vi "Iso Measurement Write.vi"(8 "error in":errorcluster, 10 "Iso Measurement STS":i32, 11 "Iso Measurement in":refnum<class "Iso Measurement.lvclass">) -> (0 "error out":errorcluster, 3 "Iso Measurement out":refnum<class "Iso Measurement.lvclass">)   [LabVIEW 2023, in "Iso Measurement.lvclass"]
uses:
  Iso Measurement.lvclass
  <vilib>/ADAS Replay HIL/Channels/Tag Wrapper/Tag Wrapper.lvlib
  <vilib>/ADAS Replay HIL/Channels/Tag Wrapper/Polymorphic/Write Channel (I32).vi
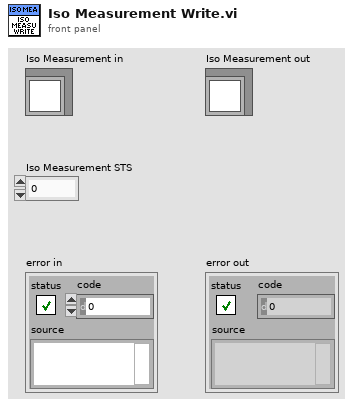
[diagram p1: front panel]
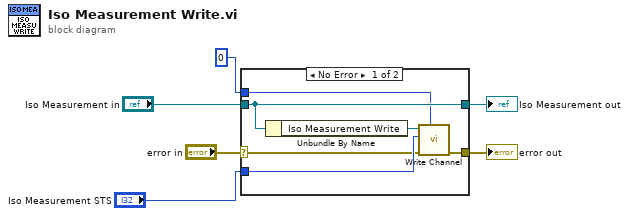
[diagram p0: block diagram]
diagram:
  n1 = case shown="No Error" "error in" {
    selector: "error in" -> [w9 w14]
    tunnel: [w8 w14] -> w5
    tunnel: [w12 w13] -> w3
    tunnel: "Iso Measurement in" -> [w12 w13]
    tunnel: "Iso Measurement STS" -> [w10 _]
    tunnel: 0 ("Timeout (ms)") -> [w7 _]
    frame No Error {
      n2 = Unbundle By Name(w12) -> ("Iso Measurement Write"=w11:refnum<k21>)
      n3 = call-poly <vilib>:"Write Channel.vi"("Timeout (ms)"=w7, "error in"=w9, "Value to Write"=w10, "ADAS HIL Channel in"=w11) -> ("error out"=w8:errorcluster)  [unwired: 5 in, 2 out]
    }
    frame Error {
    }
  }
  "error out" <- w5
  "Iso Measurement out" <- w3
